vi "Write.vi"(8 "error in (no error)":errorcluster, 10 "write buffer":string, 11 "ArduinoAISim in":refnum<class "ArduinoAISim.lvclass">) -> (0 "error out":errorcluster, 3 "ArduinoAISim out":refnum<class "ArduinoAISim.lvclass">)   [LabVIEW 2020, in "ArduinoAISim.lvclass"]
uses:
  ArduinoAISim.lvclass
  ArduinoAI/ArduinoAI.lvclass
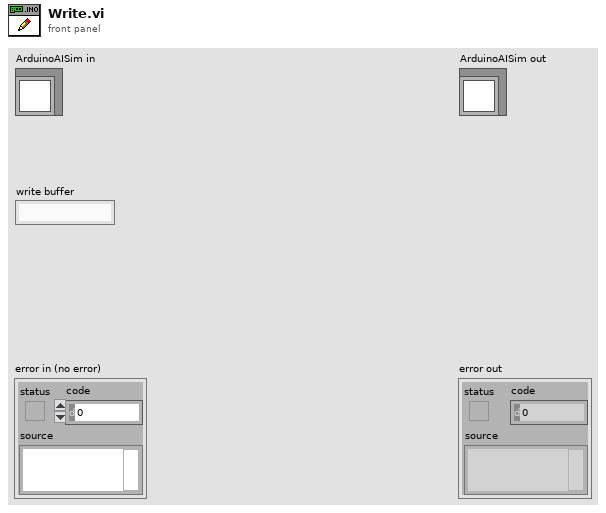
[diagram p1: front panel]
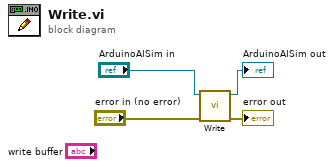
[diagram p0: block diagram]
diagram:
  n1 = call-parent "Write.vi"("error in (no error)"="error in (no error)", "ArduinoAI in"="ArduinoAISim in") -> ("error out"=→"error out":errorcluster, "ArduinoAI out"=→"ArduinoAISim out":refnum<class "ArduinoAISim.lvclass">)  [unwired: 8 in]
